vi "Bezier Curve.vi"(10 "percision":dbl, 11 "ctrl points":cluster{dbl, dbl}[](array[cluster])) -> (3 "curve":T1)   [LabVIEW 2019]
uses:
  Types/Bezier Curve.ctl
  <vilib>/Analysis/2dsp.llb/2D Inverse Complex FFT.vi
  <vilib>/Analysis/NI_AALPro.lvlib
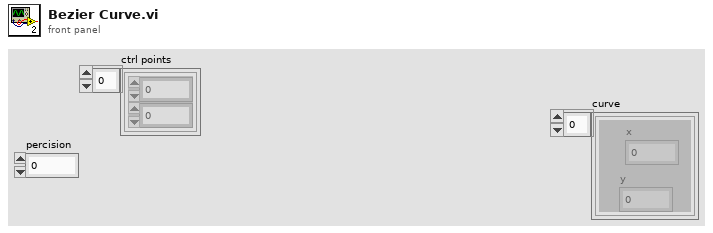
[diagram p1: front panel]
types:
  T1 = typedef "Bezier Curve.ctl" = cluster{"x":dbl, "y":dbl}[]
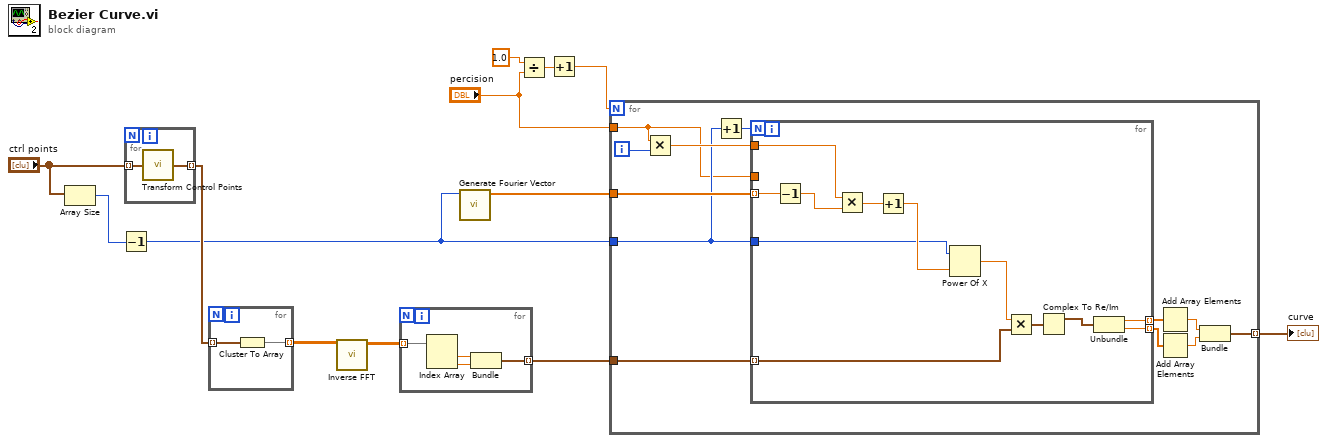
[diagram p0: block diagram]
diagram:
  n1 = Array Size(array="ctrl points") -> (size(s)=w2:i32)
  n2 = Decrement(x=w2) -> (x-1=w1:i32)
  n3 = for {
    tunnel: "ctrl points" -> [w15] mode=indexing
    tunnel: [w14] -> w5 mode=indexing
    n4 = call "Transform Control Points.vi"("ctrl pt"=w15) -> ("ctrl pt out"=w14:cluster{dbl, dbl})
  }
  n5 = for {
    tunnel: w5 -> [w17] mode=indexing
    tunnel: [w16] -> w11 mode=indexing
    n6 = Cluster To Array(cluster=w17) -> (array=w16:dbl[])
  }
  n7 = call-poly <vilib>:"Inverse FFT.vi"("FFT {x}"=w11) -> ("X"=w10:cdb[][])  [unwired: 9 in, 1 out]
  n8 = for {
    tunnel: w10 -> [w21] mode=indexing
    tunnel: [w18] -> w9 mode=indexing
    n9 = Index Array(array=w21) -> (element #1=w20:cdb, element #2=w19:cdb)  [unwired: 2 in]
    n10 = Bundle(w20, w19) -> (w18:cluster{cdb, cdb})  [unwired: 1 in]
  }
  n11 = call "Generate Fourier Vector.vi"("degree"=w1) -> ("Fourier Matrix"=w7:cdb[])  [unwired: 10 in]
  n12 = Divide(x=1.0, y="percision") -> (x/y=w4:dbl)
  n13 = Increment(x=w4) -> (x+1=w3:dbl)
  n14 = for {
    N: w3 -> [_]
    tunnel: "percision" -> [w22]
    tunnel: w1 -> [w24]
    tunnel: w9 -> [w32]
    tunnel: [w26] -> w8 mode=indexing
    tunnel: w7 -> [w25]
    i -> [w33]
    n15 = Multiply(x=w22, y=w33) -> (x*y=w31:dbl)
    n16 = Increment(x=w24) -> (x+1=w23:i32)
    n17 = for {
      N: w23 -> [_]
      tunnel: w32 -> [w38] mode=indexing
      tunnel: w24 -> [w39]
      tunnel: w31 -> [w34]
      tunnel: [w43] -> w30 mode=indexing
      tunnel: [w42] -> w29 mode=indexing
      tunnel: w25 -> [w41] mode=indexing
      tunnel: w22 -> [_]
      n18 = Decrement(x=w41) -> (x-1=w40:cdb)
      n19 = Multiply(x=w34, y=w40) -> (x*y=w45:cdb)
      n20 = Increment(x=w45) -> (x+1=w44:cdb)
      n21 = Power Of X(1:w44, 2:w39) -> (0:w37:cdb)
      n22 = Multiply(x=w37, y=w38) -> (x*y=w36:cluster{cdb, cdb})
      n23 = Complex To Re/Im(x + iy=w36) -> (x=w35:cluster{dbl, dbl})  [unwired: 1 out]
      n24 = Unbundle(w35) -> (w43:dbl, w42:dbl)
    }
    n25 = Add Array Elements(numeric array=w30) -> (sum=w27:dbl)
    n26 = Add Array Elements(numeric array=w29) -> (sum=w28:dbl)
    n27 = Bundle(w27, w28) -> (w26:cluster{dbl, dbl})  [unwired: 1 in]
  }
  "curve" <- w8
